vi "Read Turn PID.vi"() -> (3 "Cluster":T1)   [LabVIEW 2016]
uses:
  <vilib>/Rock Robotics/Network Tables/NT Read Number.vi
  <vilib>/Rock Robotics/Network Tables/NT Read Numeric Array.vi
panel:
  in  "PID":dbl[](array[numeric])
  in  "Linearity":dbl=0.6
  in  "Turn Speed":dbl=0.6
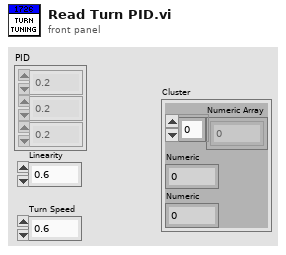
[diagram p1: front panel]
types:
  T1 = cluster{"Numeric Array":dbl[], "Numeric":dbl, "Numeric":dbl}
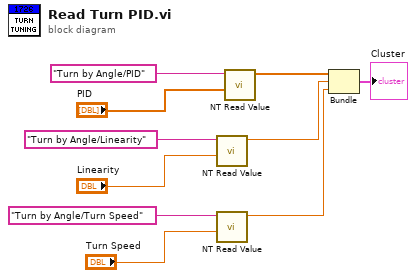
[diagram p0: block diagram]
diagram:
  n1 = call-poly <vilib>:"NT Read Value.vi"("Default Value"="Linearity", "Name"="Turn by Angle/Linearity") -> ("Numeric"=w5:dbl)  [unwired: 8 in, 1 out]
  n2 = call-poly <vilib>:"NT Read Value.vi"("Default Value"="Turn Speed", "Name"="Turn by Angle/Turn Speed") -> ("Numeric"=w6:dbl)  [unwired: 8 in, 1 out]
  n3 = call-poly <vilib>:"NT Read Value.vi"("Default Value"="PID", "Name"="Turn by Angle/PID") -> ("Numeric Array"=w4:dbl[])  [unwired: 8 in, 1 out]
  n4 = Bundle("Numeric Array"=w4, "Numeric"=w5, "Numeric"=w6) -> (→"Cluster":T1)  [unwired: 1 in]
